vi "rsidr_core_global.vi"() -> ()   [LabVIEW 2020, in "Rohde&Schwarz RTx Oscilloscopes.lvlib"] (continued)
"Write Callback"="", "Supported Models"="", "Instrument Options"="", "Flags"=0, "Help"="Sets the slope to be found on clock signal. It define the time reference point for the setup and hold time.\n\nAvailable Repeated Capabilities:\nNone\n\nRemote-control command(s):\nSEARch:TRIGger:DATatoclock:CEDGe"}, {"Level"=2, "Class Only"=FALSE, "Identifier"="RSRTX_ATTR_SEARCH_TRIGGER_D2C_SETUP_TIME", "Descriptive Name"="Search Trigger Data2Clock Setup Time", "Data Type"=1, "Command"="SEAR:TRIG:DAT:STIM", "Access"=2, "Range Table"="", "Read Callback"="", "Write Callback"="", "Supported Models"="", "Instrument Options"="", "Flags"=0, "Help"="Sets the minimum time before the clock edge while the data signal must stay steady above or below the data level. The setup time can be negative. In this case, the setup interval starts after the clock edge, and the hold time must be positive and longer than the absolute value of the setup time.\n\nAvailable Repeated Capabilities:\nNone\n\nRemote-control command(s):\nSEARch:TRIGger:DATatoclock:STIMe"}, {"Level"=2, "Class Only"=FALSE, "Identifier"="RSRTX_ATTR_SEARCH_TRIGGER_D2C_HOLD_TIME", "Descriptive Name"="Search Trigger Data2Clock Hold Time", "Data Type"=1, "Command"="SEAR:TRIG:DAT:HTIM", "Access"=2, "Range Table"="", "Read Callback"="", "Write Callback"="", "Supported Models"="", "Instrument Options"="", "Flags"=0, "Help"="Sets the minimum time after the clock edge while the data signal must stay steady above or below the data level. The hold time can be negative. In this case, the hold time ends before the clock edge, and the setup time must be positive and longer than the absolute value of the hold time.\n\nAvailable Repeated Capabilities:\nNone\n\nRemote-control command(s):\nSEARch:TRIGger:DATatoclock:HTIMe"}, {"Level"=2, "Class Only"=FALSE, "Identifier"="RSRTX_ATTR_SEARCH_TRIGGER_PATTERN", "Descriptive Name"="Search Trigger Pattern", "Data Type"=2, "Command"="SEAR:TRIG:PATT:SOUR", "Access"=2, "Range Table"="", "Read Callback"="", "Write Callback"="", "Supported Models"="", "Instrument Options"="", "Flags"=0, "Help"="Sets the state of the source channels used for pattern search.\n\nUse: 0 for Low, 1 for High, X for not matter\n\nExample: &apos;1X10&apos;\n\nNotes:\n(1) Order of channels is CH1,CH2,CH3,CH4\n\n(2) Exactly 4 channel must be specified in pattern.\n\nAvailable Repeated Capabilities:\nNone\n\nRemote-control command(s):\nSEARch:TRIGger:PATTern:SOURce"}, {"Level"=2, "Class Only"=FALSE, "Identifier"="RSRTX_ATTR_SEARCH_TRIGGER_PATTERN_COMBINATION", "Descriptive Name"="Search Trigger Pattern Combination", "Data Type"=0, "Command"="SEAR:TRIG:PATT:FUNC", "Access"=2, "Range Table"="rsrtx_rngSearchTriggerPatternCombination", "Read Callback"="", "Write Callback"="", "Supported Models"="", "Instrument Options"="", "Flags"=0, "Help"="Sets the logical combination of the channel states.\n\nAvailable Repeated Capabilities:\nNone\n\nRemote-control command(s):\nSEARch:TRIGger:PATTern:FUNCtion"}, {"Level"=2, "Class Only"=FALSE, "Identifier"="RSRTX_ATTR_SEARCH_TRIGGER_PATTERN_COMPARISON", "Descriptive Name"="Search Trigger Pattern Comparison", "Data Type"=0, "Command"="SEAR:TRIG:PATT:WIDT:RANG", "Access"=2, "Range Table"="rsrtx_rngSearchRange", "Read Callback"="", "Write Callback"="", "Supported Models"="", "Instrument Options"="", "Flags"=0, "Help"="Sets the condition how the duration of a steady pattern is compared with the given reference time.\n\nAvailable Repeated Capabilities:\nNone\n\nRemote-control command(s):\nSEARch:TRIGger:PATTern:WIDTh:RANGe"}, {"Level"=2, "Class Only"=FALSE, "Identifier"="RSRTX_ATTR_SEARCH_TRIGGER_PATTERN_WIDTH", "Descriptive Name"="Search Trigger Pattern Width", "Data Type"=1, "Command"="SEAR:TRIG:PATT:WIDT", "Access"=2, "Range Table"="", "Read Callback"="", "Write Callback"="", "Supported Models"="", "Instrument Options"="", "Flags"=0, "Help"="Sets the reference time of a steady pattern, the nominal value for comparisons.\n\nAvailable Repeated Capabilities:\nNone\n\nRemote-control command(s):\nSEARch:TRIGger:PATTern:WIDTh[:WIDTh]"}, {"Level"=2, "Class Only"=FALSE, "Identifier"="RSRTX_ATTR_SEARCH_TRIGGER_PATTERN_WIDTH_DELTA", "Descriptive Name"="Search Trigger Pattern Width Delta", "Data Type"=1, "Command"="SEAR:TRIG:PATT:WIDT:DELT", "Access"=2, "Range Table"="", "Read Callback"="", "Write Callback"="", "Supported Models"="", "Instrument Options"="", "Flags"=0, "Help"="Sets a range delta t to the reference pattern duration, when comparsion  is set to Within or Outside (see RSRTX_ATTR_SEARCH_TRIGGER_PATTERN_COMPARISON).\n\nAvailable Repeated Capabilities:\nNone\n\nRemote-control command(s):\nSEARch:TRIGger:PATTern:WIDTh:DELTa"}, {"Level"=2, "Class Only"=FALSE, "Identifier"="RSRTX_ATTR_SEARCH_TRIGGER_WINDOW_LEVEL_LOWER", "Descriptive Name"="Search Trigger Window Level Lower", "Data Type"=1, "Command"="SEAR:TRIG:LEV:WIND:LOW", "Access"=2, "Range Table"="", "Read Callback"="", "Write Callback"="", "Supported Models"="RTM|RTA", "Instrument Options"="", "Flags"=0, "Help"="Sets the voltage threshold. When the signal crosses this level, the window measurement starts or stops depending on the selected slope.\n\nAvailable Repeated Capabilities:\nNone\n\nRemote-control command(s):\nSEARch:TRIGger:LEVel:WINDow:LOWer"}, {"Level"=2, "Class Only"=FALSE, "Identifier"="RSRTX_ATTR_SEARCH_TRIGGER_WINDOW_LEVEL_UPPER", "Descriptive Name"="Search Trigger Window Level Upper", "Data Type"=1, "Command"="SEAR:TRIG:LEV:WIND:UPP", "Access"=2, "Range Table"="", "Read Callback"="", "Write Callback"="", "Supported Models"="RTM|RTA", "Instrument Options"="", "Flags"=0, "Help"="Sets the voltage threshold. When the signal crosses this level, the window measurement starts or stops depending on the selected slope.\n\nAvailable Repeated Capabilities:\nNone\n\nRemote-control command(s):\nSEARch:TRIGger:LEVel:WINDow:UPPer"}, {"Level"=2, "Class Only"=FALSE, "Identifier"="RSRTX_ATTR_SEARCH_TRIGGER_WINDOW_DELTA", "Descriptive Name"="Search Trigger Window Delta", "Data Type"=1, "Command"="SEAR:TRIG:WIND:DELT", "Access"=2, "Range Table"="", "Read Callback"="", "Write Callback"="", "Supported Models"="RTM|RTA", "Instrument Options"="", "Flags"=0, "Help"="Sets a range delta t.\n\nAvailable Repeated Capabilities:\nNone\n\nRemote-control command(s):\nSEARch:TRIGger:WINDow:DELTa"}, {"Level"=2, "Class Only"=FALSE, "Identifier"="RSRTX_ATTR_SEARCH_TRIGGER_WINDOW_POLARITY", "Descriptive Name"="Search Trigger Window Polarity", "Data Type"=0, "Command"="SEAR:TRIG:WIND:POL", "Access"=2, "Range Table"="rsrtx_rngSearchSlope", "Read Callback"="", "Write Callback"="", "Supported Models"="RTM|RTA", "Instrument Options"="", "Flags"=0, "Help"="Sets the slope to be found.\n\nAvailable Repeated Capabilities:\nNone\n\nRemote-control command(s):\nSEARch:TRIGger:WINDow:POLarity"}, {"Level"=2, "Class Only"=FALSE, "Identifier"="RSRTX_ATTR_SEARCH_TRIGGER_WINDOW_RANGE", "Descriptive Name"="Search Trigger Window Range", "Data Type"=0, "Command"="SEAR:TRIG:WIND:RANG", "Access"=2, "Range Table"="rsrtx_rngWindowRange", "Read Callback"="", "Write Callback"="", "Supported Models"="RTM|RTA", "Instrument Options"="", "Flags"=0, "Help"="Sets how the measured pulse width is compared with the given limit(s).\n\nAvailable Repeated Capabilities:\nNone\n\nRemote-control command(s):\nSEARch:TRIGger:WINDow:RANGe"}, {"Level"=2, "Class Only"=FALSE, "Identifier"="RSRTX_ATTR_SEARCH_TRIGGER_WINDOW_TIME_RANGE", "Descriptive Name"="Search Trigger Window Time Range", "Data Type"=0, "Command"="SEAR:TRIG:WIND:TIM", "Access"=2, "Range Table"="rsrtx_rngSearchRange", "Read Callback"="", "Write Callback"="", "Supported Models"="RTM|RTA", "Instrument Options"="", "Flags"=0, "Help"="Configures the window time range.\n\nAvailable Repeated Capabilities:\nNone\n\nRemote-control command(s):\nSEARch:TRIGger:WINDow:TIMerange"}, {"Level"=2, "Class Only"=FALSE, "Identifier"="RSRTX_ATTR_SEARCH_TRIGGER_WINDOW_WIDTH", "Descriptive Name"="Search Trigger Window Width", "Data Type"=1, "Command"="SEAR:TRIG:WIND:WIDT", "Access"=2, "Range Table"="", "Read Callback"="", "Write Callback"="", "Supported Models"="RTM|RTA", "Instrument Options"="", "Flags"=0, "Help"="Configures window trigger width.\n\nAvailable Repeated Capabilities:\nNone\n\nRemote-control command(s):\nSEARch:TRIGger:WINDow:WIDTh"}, {"Level"=2, "Class Only"=FALSE, "Identifier"="RSRTX_ATTR_SEARCH_GATE_MODE", "Descriptive Name"="Search Gate Mode", "Data Type"=0, "Command"="SEAR:GATE:MODE", "Access"=2, "Range Table"="rsrtx_rngSearchGateMode", "Read Callback"="", "Write Callback"="", "Supported Models"="", "Instrument Options"="", "Flags"=0, "Help"="Configures the start and end values for the gate.\n\nAvailable Repeated Capabilities:\nNone\n\nRemote-control command(s):\nSEARch:GATE:MODE"}, {"Level"=2, "Class Only"=FALSE, "Identifier"="RSRTX_ATTR_SEARCH_GATE_START", "Descriptive Name"="Search Gate Start", "Data Type"=1, "Command"="SEAR:GATE:ABS:STAR", "Access"=2, "Range Table"="", "Read Callback"="", "Write Callback"="", "Supported Models"="", "Instrument Options"="", "Flags"=0, "Help"="Sets the start time of the search area in relation to the trigger point.\n\nAvailable Repeated Capabilities:\nNone\n\nRemote-control command(s):\nSEARch:GATE:ABSolute:STARt"}, {"Level"=2, "Class Only"=FALSE, "Identifier"="RSRTX_ATTR_SEARCH_GATE_STOP", "Descriptive Name"="Search Gate Stop", "Data Type"=1, "Command"="SEAR:GATE:ABS:STOP", "Access"=2, "Range Table"="", "Read Callback"="", "Write Callback"="", "Supported Models"="", "Instrument Options"="", "Flags"=0, "Help"="Sets the stop time of the search area in relation to the trigger point.\n\nAvailable Repeated Capabilities:\nNone\n\nRemote-control command(s):\nSEARch:GATE:ABSolute:STOP"}, {"Level"=2, "Class Only"=FALSE, "Identifier"="RSRTX_ATTR_SEARCH_SHOW_RESULT", "Descriptive Name"="Search Show Result", "Data Type"=3, "Command"="SEAR:RESD:SHOW", "Access"=2, "Range Table"="", "Read Callback"="", "Write Callback"="", "Supported Models"="", "Instrument Options"="", "Flags"=0, "Help"="Shows or hides the table of search results.\n\nAvailable Repeated Capabilities:\nNone\n\nRemote-control command(s):\nSEARch:RESDiagram:SHOW"}, {"Level"=2, "Class Only"=FALSE, "Identifier"="RSRTX_ATTR_SEARCH_NUMBER_OF_RESULTS", "Descriptive Name"="Search Number Of Results", "Data Type"=0, "Command"="SEAR:RCO?", "Access"=0, "Range Table"="", "Read Callback"="", "Write Callback"="", "Supported Models"="", "Instrument Options"="", "Flags"=0, "Help"="Returns the number of search results.\n\nAvailable Repeated Capabilities:\nNone\n\nRemote-control command(s):\nSEARch:RCOunt?"}, {"Level"=2, "Class Only"=FALSE, "Identifier"="RSRTX_ATTR_SEARCH_MAXIMUM_NUMBER_OF_RESULTS", "Descriptive Name"="Search Maximum Number Of Results", "Data Type"=0, "Command"="SEAR:RES:BCO?", "Access"=0, "Range Table"="", "Read Callback"="", "Write Callback"="", "Supported Models"="", "Instrument Options"="", "Flags"=0, "Help"="Returns the maximum number of search results which the instrument can store.\n\nAvailable Repeated Capabilities:\nNone\n\nRemote-control command(s):\nSEARch:RESult:BCOunt?"}, {"Level"=2, "Class Only"=TRUE, "Identifier"="", "Descriptive Name"="Export", "Data Type"=0, "Command"="", "Access"=0, "Range Table"="", "Read Callback"="", "Write Callback"="", "Supported Models"="", "Instrument Options"="", "Flags"=0, "Help"="Contains attributes for search exporting."}, {"Level"=3, "Class Only"=FALSE, "Identifier"="RSRTX_ATTR_SEARCH_EXPORT_NAME", "Descriptive Name"="Search Export Name", "Data Type"=2, "Command"="EXP:SEAR:NAME", "Access"=2, "Range Table"="", "Read Callback"="", "Write Callback"="", "Supported Models"="", "Instrument Options"="", "Flags"=0, "Help"="Defines the path and filename of the results file, available for search. The file format is CSV. If the file already exists, it will be overwritten.\n\nAvailable Repeated Capabilities:\nNone\n\nRemote-control command(s):\nEXPort:SEARch:NAME"}, {"Level"=3, "Class Only"=FALSE, "Identifier"="RSRTX_ATTR_SEARCH_EXPORT_SAVE", "Descriptive Name"="Search Export Save", "Data Type"=4, "Command"="EXP:SEAR:SAVE", "Access"=1, "Range Table"="", "Read Callback"="", "Write Callback"="", "Supported Models"="", "Instrument Options"="", "Flags"=0, "Help"="Saves search results of the indicated measurement place to the file.\n\nAvailable Repeated Capabilities:\nNone\n\nRemote-control command(s):\nEXPort:SEARch:SAVE"}, {"Level"=2, "Class Only"=TRUE, "Identifier"="", "Descriptive Name"="Channel", "Data Type"=0, "Command"="", "Access"=0, "Range Table"="", "Read Callback"="", "Write Callback"="", "Supported Models"="", "Instrument Options"="", "Flags"=0, "Help"="Contains attributes for searching functions."}, {"Level"=3, "Class Only"=FALSE, "Identifier"="RSRTX_ATTR_SEARCH_TRIGGER_PATTERN_LEVEL", "Descriptive Name"="Search Trigger Pattern Level", "Data Type"=1, "Command"="SEAR:TRIG:PATT:LEV{Channel}", "Access"=2, "Range Table"="", "Read Callback"="", "Write Callback"="", "Supported Models"="", "Instrument Options"="", "Flags"=0, "Help"="Sets the threshold value for the selected source channel. If the signal value is higher than the trigger level, the signal state is high (1 or true for the boolean logic). Otherwise, the signal state is considered low (0 or false) if the signal value is below the trigger level.\n\nAvailable Repeated Capabilities:\nChannel: CH0, CH1, CH2, CH3, CH4, CHExt\r\n\nRemote-control command(s):\nSEARch:TRIGger:PATTern:LEVel<n>"}, {"Level"=3, "Class Only"=FALSE, "Identifier"="RSRTX_ATTR_SEARCH_TRIGGER_PATTERN_HYSTERESIS", "Descriptive Name"="Search Trigger Pattern Hysteresis", "Data Type"=1, "Command"="SEAR:TRIG:PATT:LEV{Channel}:DELT", "Access"=2, "Range Table"="", "Read Callback"="", "Write Callback"="", "Supported Models"="", "Instrument Options"="", "Flags"=0, "Help"="Sets a hysteresis range to the level of the selected source channel in order to avoid unwanted search results caused by noise oscillation around the level. For a rising edge, the hysteresis is below the search level. Otherwise, for a falling edge the hysteresis is above the level.\n\nAvailable Repeated Capabilities:\nChannel: CH0, CH1, CH2, CH3, CH4, CHExt\r\n\nRemote-control command(s):\nSEARch:TRIGger:PATTern:LEVel<n>:DELTa"}, {"Level"=2, "Class Only"=TRUE, "Identifier"="", "Descriptive Name"="LIN", "Data Type"=0, "Command"="", "Access"=0, "Range Table"="", "Read Callback"="", "Write Callback"="", "Supported Models"="", "Instrument Options"="", "Flags"=0, "Help"="Contains attributes for searching functions in LIN protocol."}, {"Level"=3, "Class Only"=FALSE, "Identifier"="RSRTX_ATTR_PROTOCOL_LIN_SEARCH_EVENT", "Descriptive Name"="Protocol LIN Search Event", "Data Type"=0, "Command"="SEAR:PROT:LIN:COND", "Access"=2, "Range Table"="rsrtx_rngProtocolSearchEvent", "Read Callback"="", "Write Callback"="", "Supported Models"="", "Instrument Options"="K3", "Flags"=0, "Help"="Sets the event or combination of events to be searched for. Depending on the selected event, further settings are required.\n\nAvailable Repeated Capabilities:\nNone\n\nRemote-control command(s):\nSEARch:PROTocol:LIN:CONDition"}, {"Level"=3, "Class Only"=FALSE, "Identifier"="RSRTX_ATTR_PROTOCOL_LIN_SEARCH_FRAME_SETUP", "Descriptive Name"="Protocol LIN Search Frame Setup", "Data Type"=0, "Command"="SEAR:PROT:LIN:FRAM", "Access"=2, "Range Table"="rsrtx_rngProtocolLINSearchFrameSetup", "Read Callback"="", "Write Callback"="", "Supported Models"="", "Instrument Options"="K3", "Flags"=0, "Help"="Selects the frame type to be searched for.\n\nAvailable Repeated Capabilities:\nNone\n\nRemote-control command(s):\nSEARch:PROTocol:LIN:FRAMe"}, {"Level"=3, "Class Only"=FALSE, "Identifier"="RSRTX_ATTR_PROTOCOL_LIN_SEARCH_CONDITION_ID", "Descriptive Name"="Protocol LIN Search Condition ID", "Data Type"=0, "Command"="SEAR:PROT:LIN:ICON", "Access"=2, "Range Table"="rsrtx_rngProtocolCondition", "Read Callback"="", "Write Callback"="", "Supported Models"="", "Instrument Options"="K3", "Flags"=0, "Help"="Sets the operator to set a specific identifier or an identifier range.\n\nAvailable Repeated Capabilities:\nNone\n\nRemote-control command(s):\nSEARch:PROTocol:LIN:ICONdition"}, {"Level"=3, "Class Only"=FALSE, "Identifier"="RSRTX_ATTR_PROTOCOL_LIN_SEARCH_CONDITION_DATA", "Descriptive Name"="Protocol LIN Search Condition Data", "Data Type"=0, "Command"="SEAR:PROT:LIN:DCON", "Access"=2, "Range Table"="rsrtx_rngProtocolCondition", "Read Callback"="", "Write Callback"="", "Supported Models"="", "Instrument Options"="K3", "Flags"=0, "Help"="Sets the operator to set a specific identifier or an identifier range.\n\nAvailable Repeated Capabilities:\nNone\n\nRemote-control command(s):\nSEARch:PROTocol:LIN:DCONdition"}, {"Level"=3, "Class Only"=FALSE, "Identifier"="RSRTX_ATTR_PROTOCOL_LIN_SEARCH_ID_PATTERN", "Descriptive Name"="Protocol LIN Search ID Pattern", "Data Type"=2, "Command"="SEAR:PROT:LIN:IDEN", "Access"=2, "Range Table"="", "Read Callback"="", "Write Callback"="", "Supported Models"="", "Instrument Options"="K3", "Flags"=0, "Help"="Defines the identifier pattern.\n\nRelevant if RSRTX_ATTR_PROTOCOL_LIN_SEARCH_EVENT is set to IDENtifier, IDData  or IDERror.\n\nAvailable Repeated Capabilities:\nNone\n\nRemote-control command(s):\nSEARch:PROTocol:LIN:IDENtifier"}, {"Level"=3, "Class Only"=FALSE, "Identifier"="RSRTX_ATTR_PROTOCOL_LIN_SEARCH_DATA_LENGTH", "Descriptive Name"="Protocol LIN Search Data Length", "Data Type"=0, "Command"="SEAR:PROT:LIN:DLEN", "Access"=2, "Range Table"="rsrtx_rngProtocolLINDataLength", "Read Callback"="", "Write Callback"="", "Supported Models"="", "Instrument Options"="K3", "Flags"=0, "Help"="Defines the length of the data pattern - the number of bytes in the pattern.\n\nAvailable Repeated Capabilities:\nNone\n\nRemote-control command(s):\nSEARch:PROTocol:LIN:DLENgth"}, {"Level"=3, "Class Only"=FALSE, "Identifier"="RSRTX_ATTR_PROTOCOL_LIN_SEARCH_DATA_PATTERN", "Descriptive Name"="Protocol LIN Search Data Pattern", "Data Type"=2, "Command"="SEAR:PROT:LIN:DATA", "Access"=2, "Range Table"="", "Read Callback"="", "Write Callback"="", "Supported Models"="", "Instrument Options"="K3", "Flags"=0, "Help"="Defines the data pattern. The pattern length is defined with RSRTX_ATTR_PROTOCOL_LIN_SEARCH_DATA_LENGTH.\n\nRelevant if RSRTX_ATTR_PROTOCOL_LIN_SEARCH_EVENT is set to IDData.\n\nAvailable Repeated Capabilities:\nNone\n\nRemote-control command(s):\nSEARch:PROTocol:LIN:DATA"}, {"Level"=3, "Class Only"=FALSE, "Identifier"="RSRTX_ATTR_PROTOCOL_LIN_SEARCH_ERROR_CHECKSUM", "Descriptive Name"="Protocol LIN Search Error Checksum", "Data Type"=3, "Command"="SEAR:PROT:LIN:CHKS", "Access"=2, "Range Table"="", "Read Callback"="", "Write Callback"="", "Supported Models"="", "Instrument Options"="K3", "Flags"=0, "Help"="Selects the error type to be searched for.\n\nAvailable Repeated Capabilities:\nNone\n\nRemote-control command(s):\nSEARch:PROTocol:LIN:CHKSerror"}, {"Level"=3, "Class Only"=FALSE, "Identifier"="RSRTX_ATTR_PROTOCOL_LIN_SEARCH_ERROR_PARITY", "Descriptive Name"="Protocol LIN Search Error Parity", "Data Type"=3, "Command"="SEAR:PROT:LIN:IPER", "Access"=2, "Range Table"="", "Read Callback"="", "Write Callback"="", "Supported Models"="", "Instrument Options"="K3", "Flags"=0, "Help"="Selects the error type to be searched for.\n\nAvailable Repeated Capabilities:\nNone\n\nRemote-control command(s):\nSEARch:PROTocol:LIN:IPERror"}, {"Level"=3, "Class Only"=FALSE, "Identifier"="RSRTX_ATTR_PROTOCOL_LIN_SEARCH_ERROR_SYNC", "Descriptive Name"="Protocol LIN Search Error Sync", "Data Type"=3, "Command"="SEAR:PROT:LIN:SYER", "Access"=2, "Range Table"="", "Read Callback"="", "Write Callback"="", "Supported Models"="", "Instrument Options"="K3", "Flags"=0, "Help"="Selects the error type to be searched for.\n\nAvailable Repeated Capabilities:\nNone\n\nRemote-control command(s):\nSEARch:PROTocol:LIN:SYERror"}, {"Level"=2, "Class Only"=TRUE, "Identifier"="", "Descriptive Name"="CAN", "Data Type"=0, "Command"="", "Access"=0, "Range Table"="", "Read Callback"="", "Write Callback"="", "Supported Models"="", "Instrument Options"="", "Flags"=0, "Help"="Contains attributes for searching functions in CAN protocol."}, {"Level"=3, "Class Only"=FALSE, "Identifier"="RSRTX_ATTR_PROTOCOL_CAN_SEARCH_EVENT", "Descriptive Name"="Protocol CAN Search Event", "Data Type"=0, "Command"="SEAR:PROT:CAN:COND", "Access"=2, "Range Table"="rsrtx_rngProtocolSearchEvent", "Read Callback"="", "Write Callback"="", "Supported Models"="", "Instrument Options"="K3", "Flags"=0, "Help"="Sets the event or combination of events to be searched for. Depending on the selected event, further settings are required.\n\nAvailable Repeated Capabilities:\nNone\n\nRemote-control command(s):\nSEARch:PROTocol:CAN:CONDition"}, {"Level"=3, "Class Only"=FALSE, "Identifier"="RSRTX_ATTR_PROTOCOL_CAN_SEARCH_FRAME_SETUP", "Descriptive Name"="Protocol CAN Search Frame Setup", "Data Type"=0, "Command"="SEAR:PROT:CAN:FRAM", "Access"=2, "Range Table"="rsrtx_rngProtocolCANSearchFrameSetup", "Read Callback"="", "Write Callback"="", "Supported Models"="", "Instrument Options"="K3", "Flags"=0, "Help"="Selects the frame type to be searched for.\n\nAvailable Repeated Capabilities:\nNone\n\nRemote-control command(s):\nSEARch:PROTocol:CAN:FRAMe"}, {"Level"=3, "Class Only"=FALSE, "Identifier"="RSRTX_ATTR_PROTOCOL_CAN_SEARCH_FRAME_TYPE", "Descriptive Name"="Protocol CAN Search Frame Type", "Data Type"=0, "Command"="SEAR:PROT:CAN:FTYP", "Access"=2, "Range Table"="rsrtx_rngProtocolCANSearchFrameType", "Read Callback"="", "Write Callback"="", "Supported Models"="", "Instrument Options"="K3", "Flags"=0, "Help"="Specifies the frame type to be searched for.\n\nAvailable Repeated Capabilities:\nNone\n\nRemote-control command(s):\nSEARch:PROTocol:CAN:FTYPe"}, {"Level"=3, "Class Only"=FALSE, "Identifier"="RSRTX_ATTR_PROTOCOL_CAN_SEARCH_ID_TYPE", "Descriptive Name"="Protocol CAN Search ID Type", "Data Type"=0, "Command"="SEAR:PROT:CAN:ITYP", "Access"=2, "Range Table"="rsrtx_rngProtocolCANIDType", "Read Callback"="", "Write Callback"="", "Supported Models"="", "Instrument Options"="K3", "Flags"=0, "Help"="Selects the format of data and remote frames.\n\nAvailable Repeated Capabilities:\nNone\n\nRemote-control command(s):\nSEARch:PROTocol:CAN:ITYPe"}, {"Level"=3, "Class Only"=FALSE, "Identifier"="RSRTX_ATTR_PROTOCOL_CAN_SEARCH_CONDITION_ID", "Descriptive Name"="Protocol CAN Search Condition ID", "Data Type"=0, "Command"="SEAR:PROT:CAN:ICON", "Access"=2, "Range Table"="rsrtx_rngProtocolCondition", "Read Callback"="", "Write Callback"="", "Supported Models"="", "Instrument Options"="K3", "Flags"=0, "Help"="Sets the operator to set a specific identifier or an identifier range.\n\nAvailable Repeated Capabilities:\nNone\n\nRemote-control command(s):\nSEARch:PROTocol:CAN:ICONdition"}, {"Level"=3, "Class Only"=FALSE, "Identifier"="RSRTX_ATTR_PROTOCOL_CAN_SEARCH_CONDITION_DATA", "Descriptive Name"="Protocol CAN Search Condition Data", "Data Type"=0, "Command"="SEAR:PROT:CAN:DCON", "Access"=2, "Range Table"="rsrtx_rngProtocolCondition", "Read Callback"="", "Write Callback"="", "Supported Models"="", "Instrument Options"="K3", "Flags"=0, "Help"="Sets the operator to set a specific identifier or an identifier range.\n\nAvailable Repeated Capabilities:\nNone\n\nRemote-control command(s):\nSEARch:PROTocol:CAN:DCONdition"}, {"Level"=3, "Class Only"=FALSE, "Identifier"="RSRTX_ATTR_PROTOCOL_CAN_SEARCH_ID_PATTERN", "Descriptive Name"="Protocol CAN Search ID Pattern", "Data Type"=2, "Command"="SEAR:PROT:CAN:IDEN", "Access"=2, "Range Table"="", "Read Callback"="", "Write Callback"="", "Supported Models"="", "Instrument Options"="K3", "Flags"=0, "Help"="Defines the identifier pattern. The pattern length is defined with RSRTX_ATTR_PROTOCOL_CAN_SEARCH_ID_TYPE.\n\nRelevant if RSRTX_ATTR_PROTOCOL_CAN_SEARCH_EVENT is set to IDENtifier, IDData, or IDERror.\n\nAvailable Repeated Capabilities:\nNone\n\nRemote-control command(s):\nSEARch:PROTocol:CAN:IDENtifier"}, {"Level"=3, "Class Only"=FALSE, "Identifier"="RSRTX_ATTR_PROTOCOL_CAN_SEARCH_DATA_LENGTH", "Descriptive Name"="Protocol CAN Search Data Length", "Data Type"=0, "Command"="SEAR:PROT:CAN:DLEN", "Access"=2, "Range Table"="rsrtx_rngProtocolCANDataLength", "Read Callback"="", "Write Callback"="", "Supported Models"="", "Instrument Options"="K3", "Flags"=0, "Help"="Defines the length of the data pattern - the number of bytes in the pattern.\n\nAvailable Repeated Capabilities:\nNone\n\nRemote-control command(s):\nSEARch:PROTocol:CAN:DLENgth"}, {"Level"=3, "Class Only"=FALSE, "Identifier"="RSRTX_ATTR_PROTOCOL_CAN_SEARCH_DATA_PATTERN", "Descriptive Name"="Protocol CAN Search Data Pattern", "Data Type"=2, "Command"="SEAR:PROT:CAN:DATA", "Access"=2, "Range Table"="", "Read Callback"="", "Write Callback"="", "Supported Models"="", "Instrument Options"="K3", "Flags"=0, "Help"="Defines the data pattern. The pattern length is defined with RSRTX_ATTR_PROTOCOL_CAN_SEARCH_DATA_LENGTH.\n\nRelevant if RSRTX_ATTR_PROTOCOL_CAN_SEARCH_EVENT is set to IDData.\n\nAvailable Repeated Capabilities:\nNone\n\nRemote-control command(s):\nSEARch:PROTocol:CAN:DATA"}, {"Level"=3, "Class Only"=FALSE, "Identifier"="RSRTX_ATTR_PROTOCOL_CAN_SEARCH_ERROR_CRC", "Descriptive Name"="Protocol CAN Search Error CRC", "Data Type"=3, "Command"="SEAR:PROT:CAN:CRC", "Access"=2, "Range Table"="", "Read Callback"="", "Write Callback"="", "Supported Models"="", "Instrument Options"="K3", "Flags"=0, "Help"="Selects the error type to be searched for.\n\nAvailable Repeated Capabilities:\nNone\n\nRemote-control command(s):\nSEARch:PROTocol:CAN:CRCerror"}, {"Level"=3, "Class Only"=FALSE, "Identifier"="RSRTX_ATTR_PROTOCOL_CAN_SEARCH_ERROR_STUFFING", "Descriptive Name"="Protocol CAN Search Error Stuffing", "Data Type"=3, "Command"="SEAR:PROT:CAN:BITS", "Access"=2, "Range Table"="", "Read Callback"="", "Write Callback"="", "Supported Models"="", "Instrument Options"="K3", "Flags"=0, "Help"="Selects the error type to be searched for.\n\nAvailable Repeated Capabilities:\nNone\n\nRemote-control command(s):\nSEARch:PROTocol:CAN:BITSerror"}, {"Level"=3, "Class Only"=FALSE, "Identifier"="RSRTX_ATTR_PROTOCOL_CAN_SEARCH_ERROR_FORM", "Descriptive Name"="Protocol CAN Search Error Form", "Data Type"=3, "Command"="SEAR:PROT:CAN:FORM", "Access"=2, "Range Table"="", "Read Callback"="", "Write Callback"="", "Supported Models"="", "Instrument Options"="K3", "Flags"=0, "Help"="Selects the error type to be searched for.\n\nAvailable Repeated Capabilities:\nNone\n\nRemote-control command(s):\nSEARch:PROTocol:CAN:FORMerror"}, {"Level"=3, "Class Only"=FALSE, "Identifier"="RSRTX_ATTR_PROTOCOL_CAN_SEARCH_ERROR_ACK", "Descriptive Name"="Protocol CAN Search Error Ack", "Data Type"=3, "Command"="SEAR:PROT:CAN:ACK", "Access"=2, "Range Table"="", "Read Callback"="", "Write Callback"="", "Supported Models"="", "Instrument Options"="K3", "Flags"=0, "Help"="Selects the error type to be searched for.\n\nAvailable Repeated Capabilities:\nNone\n\nRemote-control command(s):\nSEARch:PROTocol:CAN:ACKerror"}, {"Level"=2, "Class Only"=TRUE, "Identifier"="", "Descriptive Name"="MILSTD", "Data Type"=0, "Command"="", "Access"=0, "Range Table"="", "Read Callback"="", "Write Callback"="", "Supported Models"="", "Instrument Options"="", "Flags"=0, "Help"="The MIL-STD-1553 specification defines the characteristics of a serial data bus originally designed for use in the military avionics. Nowadays it is also used in spacecraft on-board data handling."}, {"Level"=3, "Class Only"=FALSE, "Identifier"="RSRTX_ATTR_MILSTD_SEARCH_CONDITION", "Descriptive Name"="MILSTD Search Condition", "Data Type"=0, "Command"="SEAR:PROT:MILS:COND", "Access"=2, "Range Table"="rsrtx_rngMILSTDSearchCondition", "Read Callback"="", "Write Callback"="", "Supported Models"="RTM|RTA", "Instrument Options"="", "Flags"=0, "Help"="Selects the condition to be searched for.\n\nAvailable Repeated Capabilities:\nNone\n\nRemote-control command(s):\nSEARch:PROTocol:MILStd:CONDition"}, {"Level"=3, "Class Only"=FALSE, "Identifier"="RSRTX_ATTR_MILSTD_SEARCH_WORD_START", "Descriptive Name"="MILSTD Search Word Start", "Data Type"=0, "Command"="SEAR:PROT:MILS:WST", "Access"=2, "Range Table"="rsrtx_rngMILSTDSearchWordStart", "Read Callback"="", "Write Callback"="", "Supported Models"="RTM|RTA", "Instrument Options"="", "Flags"=0, "Help"="Selects a word start to be searched for.\n\nAvailable Repeated Capabilities:\nNone\n\nRemote-control command(s):\nSEARch:PROTocol:MILStd:WSTart"}, {"Level"=3, "Class Only"=FALSE, "Identifier"="RSRTX_ATTR_MILSTD_SEARCH_ERROR", "Descriptive Name"="MILSTD Search Error", "Data Type"=0, "Command"="SEAR:PROT:MILS:ERR", "Access"=2, "Range Table"="rsrtx_rngMILSTDSearchError", "Read Callback"="", "Write Callback"="", "Supported Models"="RTM|RTA", "Instrument Options"="", "Flags"=0, "Help"="Selects the error type to be searched for.\n\nAvailable Repeated Capabilities:\nNone\n\nRemote-control command(s):\nSEARch:PROTocol:MILStd:ERRor"}, {"Level"=3, "Class Only"=FALSE, "Identifier"="RSRTX_ATTR_MILSTD_SEARCH_TRANSMISSION_TYPE", "Descriptive Name"="MILSTD Search Transmission Type", "Data Type"=0, "Command"="SEAR:PROT:MILS:TTYP", "Access"=2, "Range Table"="rsrtx_rngMILSTDTransmissionType", "Read Callback"="", "Write Callback"="", "Supported Models"="RTM|RTA", "Instrument Options"="", "Flags"=0, "Help"="Selects the transmission type to be searched for.\n\nAvailable Repeated Capabilities:\nNone\n\nRemote-control command(s):\nSEARch:PROTocol:MILStd:TTYPe"}, {"Level"=3, "Class Only"=TRUE, "Identifier"="", "Descriptive Name"="Command", "Data Type"=0, "Command"="", "Access"=0, "Range Table"="", "Read Callback"="", "Write Callback"="", "Supported Models"="", "Instrument Options"="", "Flags"=0, "Help"="Searches on a command word."}, {"Level"=4, "Class Only"=FALSE, "Identifier"="RSRTX_ATTR_MILSTD_SEARCH_COMMAND_DATA_DIRECTION", "Descriptive Name"="MILSTD Search Command Data Direction", "Data Type"=0, "Command"="SEAR:PROT:MILS:TRM", "Access"=2, "Range Table"="rsrtx_rngMILSTDDirection", "Read Callback"="", "Write Callback"="", "Supported Models"="RTM|RTA", "Instrument Options"="", "Flags"=0, "Help"="Selects the transmission mode to be searched for.\n\nAvailable Repeated Capabilities:\nNone\n\nRemote-control command(s):\nSEARch:PROTocol:MILStd:TRMode"}, {"Level"=4, "Class Only"=FALSE, "Identifier"="RSRTX_ATTR_MILSTD_SEARCH_RT_ADDRESS_CONDITION", "Descriptive Name"="MILSTD Search RT Address Condition", "Data Type"=0, "Command"="SEAR:PROT:MILS:RTAD:COND", "Access"=2, "Range Table"="rsrtx_rngMILSTDCondition", "Read Callback"="", "Write Callback"="", "Supported Models"="RTM|RTA", "Instrument Options"="", "Flags"=0, "Help"="For an RT address, searches for a comparison condition.\n\nAvailable Repeated Capabilities:\nNone\n\nRemote-control command(s):\nSEARch:PROTocol:MILStd:RTADdress:CONDition"}, {"Level"=4, "Class Only"=FALSE, "Identifier"="RSRTX_ATTR_MILSTD_SEARCH_RT_ADDRESS_MINIMUM", "Descriptive Name"="MILSTD Search RT Address Minimum", "Data Type"=2, "Command"="SEAR:PROT:MILS:RTAD:MIN", "Access"=2, "Range Table"="", "Read Callback"="", "Write Callback"="", "Supported Models"="RTM|RTA", "Instrument Options"="", "Flags"=0, "Help"="For an RT address, searches for the minimum address.\n01X-string\n\nAvailable Repeated Capabilities:\nNone\n\nRemote-control command(s):\nSEARch:PROTocol:MILStd:RTADdress:MINimum"}, {"Level"=4, "Class Only"=FALSE, "Identifier"="RSRTX_ATTR_MILSTD_SEARCH_RT_ADDRESS_MAXIMUM", "Descriptive Name"="MILSTD Search RT Address Maximum", "Data Type"=2, "Command"="SEAR:PROT:MILS:RTAD:MAX", "Access"=2, "Range Table"="", "Read Callback"="", "Write Callback"="", "Supported Models"="RTM|RTA", "Instrument Options"="", "Flags"=0, "Help"="For an RT address, searches for the maximum address.\n01X-string\n\nAvailable Repeated Capabilities:\nNone\n\nRemote-control command(s):\nSEARch:PROTocol:MILStd:RTADdress:MAXimum"}, {"Level"=4, "Class Only"=FALSE, "Identifier"="RSRTX_ATTR_MILSTD_SEARCH_SUB_ADDRESS_CONDITION", "Descriptive Name"="MILSTD Search Sub Address Condition", "Data Type"=0, "Command"="SEAR:PROT:MILS:SADD:COND", "Access"=2, "Range Table"="rsrtx_rngMILSTDCondition", "Read Callback"="", "Write Callback"="", "Supported Models"="RTM|RTA", "Instrument Options"="", "Flags"=0, "Help"="For the sub address, sets the triggering condition for the comparison of the decoded value to the defined range.\n\nAvailable Repeated Capabilities:\nNone\n\nRemote-control command(s):\nSEARch:PROTocol:MILStd:SADDress:CONDition"}, {"Level"=4, "Class Only"=FALSE, "Identifier"="RSRTX_ATTR_MILSTD_SEARCH_SUB_ADDRESS_MINIMUM", "Descriptive Name"="MILSTD Search Sub Address Minimum", "Data Type"=2, "Command"="SEAR:PROT:MILS:SADD:MIN", "Access"=2, "Range Table"="", "Read Callback"="", "Write Callback"="", "Supported Models"="RTM|RTA", "Instrument Options"="", "Flags"=0, "Help"="For a subaddress, searches for the minimum address.\n01X-string\n\nAvailable Repeated Capabilities:\nNone\n\nRemote-control command(s):\nSEARch:PROTocol:MILStd:SADDress:MINimum"}, {"Level"=4, "Class Only"=FALSE, "Identifier"="RSRTX_ATTR_MILSTD_SEARCH_SUB_ADDRESS_MAXIMUM", "Descriptive Name"="MILSTD Search Sub Address Maximum", "Data Type"=2, "Command"="SEAR:PROT:MILS:SADD:MAX", "Access"=2, "Range Table"="", "Read Callback"="", "Write Callback"="", "Supported Models"="RTM|RTA", "Instrument Options"="", "Flags"=0, "Help"="For a subaddress, searches for the maximum address.\n01X-string\n\nAvailable Repeated Capabilities:\nNone\n\nRemote-control command(s):\nSEARch:PROTocol:MILStd:SADDress:MAXimum"}, {"Level"=4, "Class Only"=FALSE, "Identifier"="RSRTX_ATTR_MILSTD_SEARCH_SUB_ADDRESS", "Descriptive Name"="MILSTD Search Sub Address", "Data Type"=0, "Command"="SEAR:PROT:MILS:SADD:MCAD", "Access"=2, "Range Table"="rsrtx_rngMILSTDSubAddress", "Read Callback"="", "Write Callback"="", "Supported Models"="RTM|RTA", "Instrument Options"="", "Flags"=0, "Help"="Searches for a mode code address.\n\nAvailable Repeated Capabilities:\nNone\n\nRemote-control command(s):\nSEARch:PROTocol:MILStd:SADDress:MCADdress"}, {"Level"=4, "Class Only"=FALSE, "Identifier"="RSRTX_ATTR_MILSTD_SEARCH_WORD_CONDITION", "Descriptive Name"="MILSTD Search Word Condition", "Data Type"=0, "Command"="SEAR:PROT:MILS:WCO:COND", "Access"=2, "Range Table"="rsrtx_rngMILSTDCondition", "Read Callback"="", "Write Callback"="", "Supported Models"="RTM|RTA", "Instrument Options"="", "Flags"=0, "Help"="For a command word, triggers on a word comparison condition.\n\nAvailable Repeated Capabilities:\nNone\n\nRemote-control command(s):\nSEARch:PROTocol:MILStd:WCOunt:CONDition"}, {"Level"=4, "Class Only"=FALSE, "Identifier"="RSRTX_ATTR_MILSTD_SEARCH_WORD_MINIMUM", "Descriptive Name"="MILSTD Search Word Minimum", "Data Type"=0, "Command"="SEAR:PROT:MILS:WCO:MIN", "Access"=2, "Range Table"="", "Read Callback"="", "Write Callback"="", "Supported Models"="RTM|RTA", "Instrument Options"="", "Flags"=0, "Help"="Searches for the minimum word count.\n01X-string\n\nAvailable Repeated Capabilities:\nNone\n\nRemote-control command(s):\nSEARch:PROTocol:MILStd:WCOunt:MINimum"}, {"Level"=4, "Class Only"=FALSE, "Identifier"="RSRTX_ATTR_MILSTD_SEARCH_WORD_MAXIMUM", "Descriptive Name"="MILSTD Search Word Maximum", "Data Type"=0, "Command"="SEAR:PROT:MILS:WCO:MAX", "Access"=2, "Range Table"="", "Read Callback"="", "Write Callback"="", "Supported Models"="RTM|RTA", "Instrument Options"="", "Flags"=0, "Help"="Searches for the maximum word count.\n01X-string\n\nAvailable Repeated Capabilities:\nNone\n\nRemote-control command(s):\nSEARch:PROTocol:MILStd:WCOunt:MAXimum"}, {"Level"=4, "Class Only"=FALSE, "Identifier"="RSRTX_ATTR_MILSTD_SEARCH_COMMAND_MODE_CODE", "Descriptive Name"="MILSTD Search Command Mode Code", "Data Type"=0, "Command"="SEAR:PROT:MILS:MCOD", "Access"=2, "Range Table"="rsrtx_rngMILSTDCodeType", "Read Callback"="", "Write Callback"="", "Supported Models"="RTM|RTA", "Instrument Options"="", "Flags"=0, "Help"="Searches for a mode code type.\n\nAvailable Repeated Capabilities:\nNone\n\nRemote-control command(s):\nSEARch:PROTocol:MILStd:MCODe"}, {"Level"=3, "Class Only"=TRUE, "Identifier"="", "Descriptive Name"="Status", "Data Type"=0, "Command"="", "Access"=0, "Range Table"="", "Read Callback"="", "Write Callback"="", "Supported Models"="", "Instrument Options"="", "Flags"=0, "Help"="Searches for a status word that is specified."}, {"Level"=4, "Class Only"=FALSE, "Identifier"="RSRTX_ATTR_MILSTD_SEARCH_RECEIVED_BIT_STATUS", "Descriptive Name"="MILSTD Search Received Bit Status", "Data Type"=0, "Command"="SEAR:PROT:MILS:STAT:BCR", "Access"=2, "Range Table"="rsrtx_rngStatus", "Read Callback"="", "Write Callback"="", "Supported Models"="RTM|RTA", "Instrument Options"="", "Flags"=0, "Help"="Searches for a broadcast received bit of a status word.\n01X-string\n\nAvailable Repeated Capabilities:\nNone\n\nRemote-control command(s):\nSEARch:PROTocol:MILStd:STATus:BCReceived"}, {"Level"=4, "Class Only"=FALSE, "Identifier"="RSRTX_ATTR_MILSTD_SEARCH_BUSY_BIT_STATUS", "Descriptive Name"="MILSTD Search Busy Bit Status", "Data Type"=0, "Command"="SEAR:PROT:MILS:STAT:BUSY", "Access"=2, "Range Table"="rsrtx_rngStatus", "Read Callback"="", "Write Callback"="", "Supported Models"="RTM|RTA", "Instrument Options"="", "Flags"=0, "Help"="Searches for a busy bit of a status word.\n01X-string\n\nAvailable Repeated Capabilities:\nNone\n\nRemote-control command(s):\nSEARch:PROTocol:MILStd:STATus:BUSY"}, {"Level"=4, "Class Only"=FALSE, "Identifier"="RSRTX_ATTR_MILSTD_SEARCH_BUS_CONTROL_BIT_STATUS", "Descriptive Name"="MILSTD Search Bus Control Bit Status", "Data Type"=0, "Command"="SEAR:PROT:MILS:STAT:DBC", "Access"=2, "Range Table"="rsrtx_rngStatus", "Read Callback"="", "Write Callback"="", "Supported Models"="RTM|RTA", "Instrument Options"="", "Flags"=0, "Help"="Searches for a dynamic bus control accept bit of a status word.\n01X-string\n\nAvailable Repeated Capabilities:\nNone\n\nRemote-control command(s):\nSEARch:PROTocol:MILStd:STATus:DBCaccept"}, {"Level"=4, "Class Only"=FALSE, "Identifier"="RSRTX_ATTR_MILSTD_SEARCH_INSTRUMENTATION_BIT_STATUS", "Descriptive Name"="MILSTD Search Instrumentation Bit Status", "Data Type"=0, "Command"="SEAR:PROT:MILS:STAT:INST", "Access"=2, "Range Table"="rsrtx_rngStatus", "Read Callback"="", "Write Callback"="", "Supported Models"="RTM|RTA", "Instrument Options"="", "Flags"=0, "Help"="Searches for an instrument bit of a status word.\n01X-string\n\nAvailable Repeated Capabilities:\nNone\n\nRemote-control command(s):\nSEARch:PROTocol:MILStd:STATus:INSTrument"}, {"Level"=4, "Class Only"=FALSE, "Identifier"="RSRTX_ATTR_MILSTD_SEARCHMESSAGE_ERROR_BIT_STATUS", "Descriptive Name"="MILSTD SearchMessage Error Bit Status", "Data Type"=0, "Command"="SEAR:PROT:MILS:STAT:MERR", "Access"=2, "Range Table"="rsrtx_rngStatus", "Read Callback"="", "Write Callback"="", "Supported Models"="RTM|RTA", "Instrument Options"="", "Flags"=0, "Help"="Searches for a message error bit of a status word.\n01X-string\n\nAvailable Repeated Capabilities:\nNone\n\nRemote-control command(s):\nSEARch:PROTocol:MILStd:STATus:MERRor"}, {"Level"=4, "Class Only"=FALSE, "Identifier"="RSRTX_ATTR_MILSTD_SEARCH_SERVICE_REQUEST_BIT_STATUS", "Descriptive Name"="MILSTD Search Service Request Bit Status", "Data Type"=0, "Command"="SEAR:PROT:MILS:STAT:SREQ", "Access"=2, "Range Table"="rsrtx_rngStatus", "Read Callback"="", "Write Callback"="", "Supported Models"="RTM|RTA", "Instrument Options"="", "Flags"=0, "Help"="Searches for a service request bit of a status word.\n01X-string\n\nAvailable Repeated Capabilities:\nNone\n\nRemote-control command(s):\nSEARch:PROTocol:MILStd:STATus:SREQuest"}, {"Level"=4, "Class Only"=FALSE, "Identifier"="RSRTX_ATTR_MILSTD_SEARCH_SUBSYSTEM_BIT_STATUS", "Descriptive Name"="MILSTD Search Subsystem Bit Status", "Data Type"=0, "Command"="SEAR:PROT:MILS:STAT:SUBS", "Access"=2, "Range Table"="rsrtx_rngStatus", "Read Callback"="", "Write Callback"="", "Supported Models"="RTM|RTA", "Instrument 
